vi "Get Project Types.vi"(10 "Project:Active Project":refnum<vi>) -> (1 "All Type Name Library File Path":T1, 2 "Project Type Name Library File Path":T1)   [LabVIEW 2020, in "_Shared.lvlib"]
uses:
  _Shared.lvlib
  jettl/jettl/Msg/Msg.lvclass
  jettl/jettl/Actor/Actor.lvclass
  Name Library File Path.ctl
  Type.ctl
  Type Name Library File Path.ctl
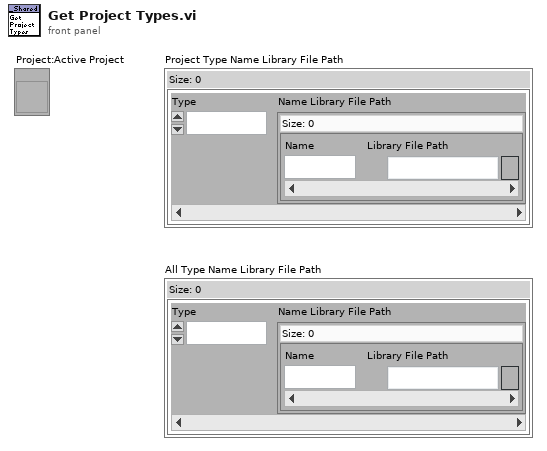
[diagram p1: front panel]
types:
  T1 = typedef "_Shared.lvlib/Type Name Library File Path.ctl" = map{T2, T3}
  T2 = typedef "_Shared.lvlib/Type.ctl" = enum16{"Actor", "Msg"}
  T3 = typedef "_Shared.lvlib/Name Library File Path.ctl" = map{string, path}
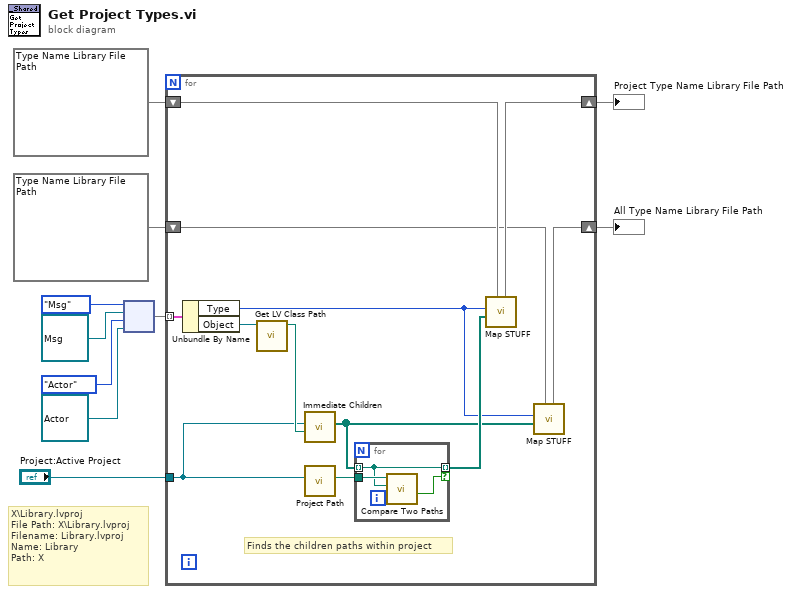
[diagram p0: block diagram]
diagram:
  # "X\\Library.lvproj\nFile Path: X\\Library.lvproj\nFilename: Library.lvproj\nName: Library\nPath: X"
  n1 = node(Type."Msg" ("Type"), refnum<class "Msg.lvclass"> refnum ("Object"), Type."Actor" ("Type"), refnum<class "Actor.lvclass"> refnum ("jettl.lvlib:Actor.lvlib:Actor.lvclass")) -> (w3:map{T2, refnum<class>})
  n2 = for {
    shift-right: [w18] -> w8
    shift-left: T1 {} ("Type Name Library File Path") -> [w22]
    tunnel: "Project:Active Project" -> [w20]
    tunnel: w3 -> [w16] mode=indexing
    shift-right: [w13] -> w1
    shift-left: T1 {} ("Type Name Library File Path") -> [w14]
    # "Finds the children paths within project"
    n3 = Unbundle By Name(w16) -> ("Type"=w12:T2, "Object"=w15:refnum<class>)
    n4 = call <vilib>:"Get LV Class Path.vi"("object"=w15) -> ("class path"=w21:path)  [unwired: 9 in, 1 out]
    n5 = call "Immediate Children.vi"("Type File Path"=w21, "Project:Active Project"=w20) -> ("Implemented Class File Paths"=w11:path[])  [unwired: 8 in, 1 out]
    n6 = call "Project Path.vi"("Project:Active Project"=w20) -> ("Project Path"=w19:path)  [unwired: 10 in]
    n7 = for {
      tunnel: w11 -> [w23] mode=indexing
      tunnel: [w23] -> w17 mode=indexing if=w25
      tunnel: w19 -> [w24]
      n8 = call <vilib>:"Compare Two Paths.vi"("Path 2"=w23, "Path 1"=w24) -> ("Path 2 Relative to Path 1?"=w25:bool)  [unwired: 6 in, 3 out]
    }
    n9 = call "Map STUFF.vi"("Type Name Library File Path in"=w22, "Implemented Class File Paths"=w17, "Type"=w12) -> ("Type Name Library File Path out"=w18:T1)  [unwired: 8 in]
    n10 = call "Map STUFF.vi"("Type Name Library File Path in"=w14, "Implemented Class File Paths"=w11, "Type"=w12) -> ("Type Name Library File Path out"=w13:T1)  [unwired: 8 in]
  }
  "Project Type Name Library File Path" <- w8
  "All Type Name Library File Path" <- w1
